vi "Rudyk2.vi"(0 "VISA resource name":refnum<visa-resource-name>="COM1", 1 "baud rate":u32=9600, 2 "data bits":u16=8 min=5 max=8 step=1, 3 "parity":u16(ring) items=["None", "Odd", "Even", "Mark", "Space"], 4 "stop bits":u16(ring)=10 items=["1.0"=10, "1.5"=15, "2.0"=20], 7 "flow control":u16(ring) items=["None"=0, "XON/XOFF"=1, "RTS/CTS"=2, "DTR/DSR"=4]) -> ()   [LabVIEW 2017]
doc: "The Basic Serial Read and Write example performs a Serial Port Read, a Serial Port Write, or a combination of these actions. The user selects the actions (read or write) on the front panel. If both are selected, the VI will write the data first, read data, and then close the VISA session that is opened to the port. This VI will wait until the specified number of bytes is received at the port. Only the number of bytes specified will be read.\n\nINSTRUCTIONS:\n1) Select the serial resource and configuration parameters (baud rate, data bits, parity, stop bits, flow control).\n2) Select the operations to be performed. \n3) Connect the serial port to your device. If no device is available, perform a loopback test by doing one of the following. Short pins 2 and 3 on a RS-232 cable or short pin 4 to pin 8 and pin 5 to pin 9 on a RS-485/422 cable. \n4) Run the VI to see the data read. (The \"read string\" will match the \"string to write\" if a loopback test was performed.)\n\nNote: The parameters set for the serial port must match the parameters of the connected instrument or device. In this example, the bytes to read parameter specifies the number of bytes that the serial port reads. If there were more bytes at the port than the number specified in bytes to read, those bytes would not be read. Also, if you specify to read more bytes than the number of bytes actually read, you might receive a timeout error message.\n\nOn the block diagram, the Configure Serial Port VI sets the configuration parameters. The front panel displays the controls used to configure the basic parameters, such as baud rate, data bits, and parity. Constants configure the other parameters the user probably does not need set. After the VISA Configure Serial Port VI opens the VISA session and configures the port, the VI passes the VISA resource name to other VIs that perform operations on that VISA resource. The VISA Write function sends a command to the serial device and the VISA Read function returns data based on the command. The VISA Close function then closes the reference to the serial device. It is important to close the reference; otherwise communication through with that port through protocols other than VISA might not be possible."
uses:
  <vilib>/Instr/_visa.llb/VISA Configure Serial Port (Instr).vi
  <vilib>/Utility/file.llb/Write To Spreadsheet File (DBL).vi
panel:
  out "Waveform Chart":dbl(graph)
  out "srednia":string
  out "read string":string
  out "bytes read":u32
  in  "delay before read (ms)":u32=500
  in  "string to write":string="*IDN?\r\n"
  in  "write":bool=TRUE
  in  "stop":bool
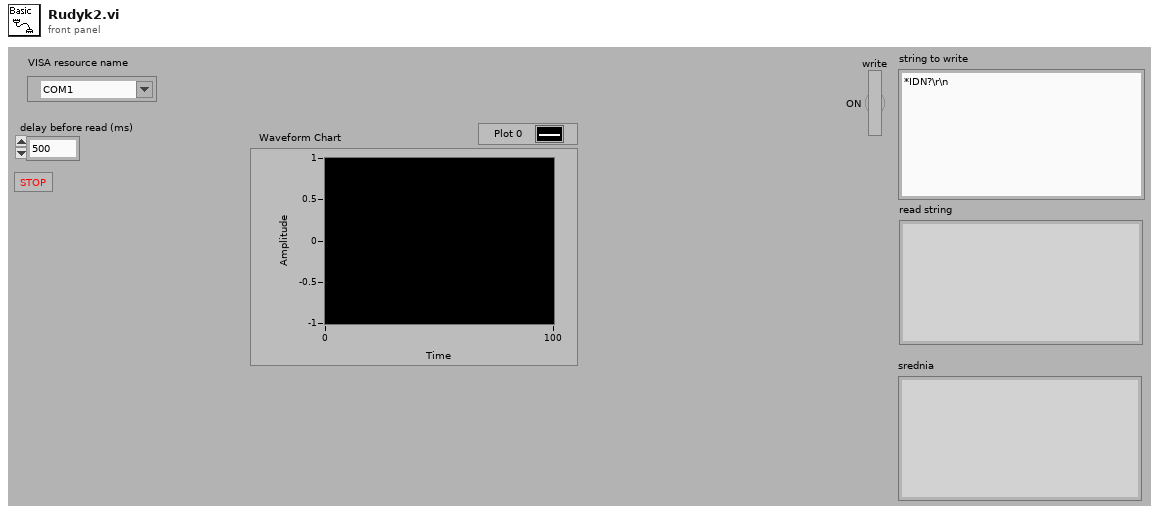
[diagram p1: front panel]
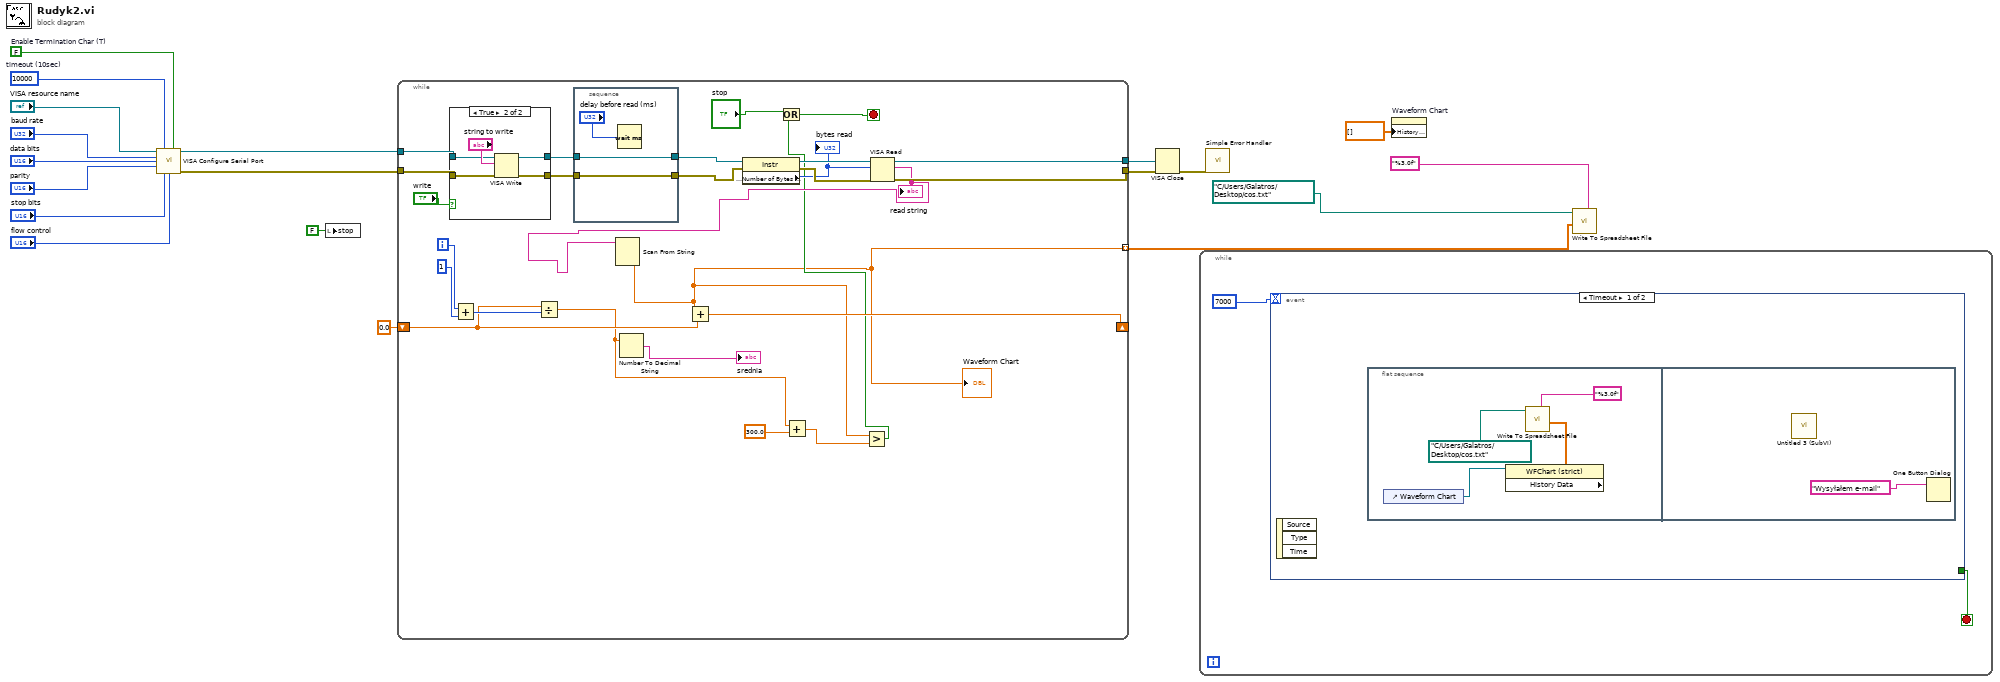
[diagram p0: block diagram]
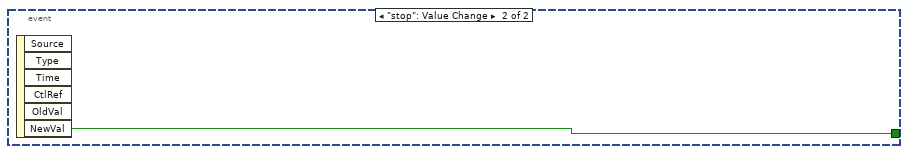
[diagram p2: hidden frame]
diagram:
  w14 = FALSE  # Enable Termination Char (T)
  w15 = u32 10000  # timeout (10sec)
  n1 = call-poly "VISA Configure Serial Port"("VISA resource name"="VISA resource name", "timeout (10sec)"=w15, "Enable Termination\nChar (T)"=w14, "baud rate (9600)"="baud rate", "data bits (8)"="data bits", "parity (0:none)"="parity", "stop bits (10: 1 bit)"="stop bits", "flow control (0:none)"="flow control") -> ("VISA resource name out"=w10:refnum<visa-resource-name>, "error out"=w9:errorcluster)  [unwired: 6 in]
  n2 = local write "stop"(FALSE ("stop")) -> ()
  n3 = while {
    tunnel: w10 -> [w37]
    tunnel: w9 -> [w36]
    tunnel: [w34] -> w7
    tunnel: [w35] -> w8
    shift-right: [w33] -> _
    shift-left: 0.0 -> [w28]
    tunnel: [w20] -> w2 mode=indexing
    i -> [w32]
    stop <- w21 stop-if-true
    n4 = case shown="True" "write" {
      tunnel: [w50 w55] -> w44
      tunnel: w37 -> [w49 w53]
      tunnel: w36 -> [w50 w52]
      tunnel: [w49 w51] -> w43
      frame False {
      }
      frame True {
        n5 = VISA Write(VISA resource name=w53, write buffer="string to write", error in (no error)=w52) -> (VISA resource name out=w51:refnum<visa-resource-name>, error out=w55:errorcluster)  [unwired: 1 out]
      }
    }
    n6 = Add(x=w32, y=1) -> (x+y=w30:i32)
    n7 = Divide(x=w28, y=w30) -> (x/y=w24:dbl)
    n8 = stacked-sequence {
      tunnel: w44 -> [w48]
      tunnel: [w48] -> w41
      tunnel: w43 -> [w47]
      tunnel: [w47] -> w42
      frame #0 {
        n9 = Wait (ms)(milliseconds to wait="delay before read (ms)") -> ()  [unwired: 1 out]
      }
    }
    n10 = Number To Decimal String(number=w24) -> (decimal integer string=→"srednia":string)  [unwired: 1 in]
    n11 = property class="Instr"(reference=w42, error in=w41) -> (reference out=w40:refnum<visa-resource-name>, error out=w39:errorcluster, "Serial Settings:Number of Bytes at Serial Port"=w38:u32)
    "bytes read" <- w38
    n12 = Add(x=w24, y=300.0) -> (x+y=w25:dbl)
    n13 = VISA Read(VISA resource name=w40, byte count=w38, error in (no error)=w39) -> (VISA resource name out=w35:refnum<visa-resource-name>, read buffer=w27:string, error out=w34:errorcluster)  [unwired: 1 out]
    "read string" <- w27
    n14 = Scan From String(input string=w27) -> (output 1=w20:dbl)  [unwired: 4 in, 3 out]
    "Waveform Chart" <- w20
    n15 = Add(x=w20, y=w28) -> (x+y=w33:dbl)
    n16 = Greater?(x=w20, y=w25) -> (0:w23:bool)
    n17 = Or(x="stop", y=w23) -> (x .or. y?=w21:bool)
  }
  n18 = VISA Close(VISA resource name=w8, error in (no error)=w7) -> (error out=w17:errorcluster)
  n19 = while {
    stop <- w56 stop-if-true
    n20 = event shown="[0] Timeout" {
      selector: _ -> [_ _]
      dyn-events: _ -> [_ _]
      timeout: 7000 -> [_ _]
      tunnel: [_ w63] -> w56
      event Timeout {
        n21 = event-data() -> ()  [unwired: 1 in, 3 out]
        n22 = flat-sequence {
          frame #0 {
            n23 = control-ref of="Waveform Chart"() -> (w59:refnum<vi>)
            n24 = property on="Property Node" class="WFChart (strict)"(reference=w59) -> ("History Data"=w60:dbl[])  [unwired: 1 in, 2 out]
            n25 = call-poly <vilib>:"Write To Spreadsheet File.vi"("format (%.3f)"="%3.0f", "1D data"=w60, "file path (dialog if empty)"=path "C:/Users/Galatros/Desktop/cos.txt" ("Path")) -> ()  [unwired: 5 in, 1 out]
          }
          frame #1 {
            n26 = call "Untitled 3 (SubVI).vi"() -> ()  [unwired: 12 in]
            n27 = One Button Dialog(message="Wysyłałem e-mail") -> ()  [unwired: 1 in, 1 out]
          }
        }
      }
      event "stop": Value Change {
        n28 = event-data() -> ("NewVal"=w63:bool)  [unwired: 1 in, 5 out]
      }
    }
  }
  n29 = call <vilib>:"Simple Error Handler.vi"("error in (no error)"=w17) -> ()  [unwired: 4 in, 5 out]
  n30 = property on="Waveform Chart" class="WFChart (strict)"("History Data"=dbl[] []) -> ()  [unwired: 2 in, 2 out]
  n31 = call-poly <vilib>:"Write To Spreadsheet File.vi"("format (%.3f)"="%3.0f", "1D data"=w2, "file path (dialog if empty)"=path "C:/Users/Galatros/Desktop/cos.txt" ("Path")) -> ()  [unwired: 5 in, 1 out]
